vi "SphereWedgeSection.vi"(0 "Ducer":cluster{"radius":dbl, "h":dbl, "a":dbl} {"radius" format="%.2f"; "a" format="%.2f"; "h" format="%.2f"}, 2 "Rotate":dbl format="%.2f") -> (1 "thetas":dbl[](array[numeric]) format="%.2f", 4 "phis":dbl[](array[numeric]) format="%.2f", 6 "x matrix":dbl[][](array[numeric]) format="%.2f", 7 "y matrix":dbl[][](array[numeric]) format="%.2f", 8 "z matrix":dbl[][](array[numeric]) format="%.2f")   [LabVIEW 2022 SP3]
uses:
  <vilib>/Analysis/NI_AALPro.lvlib
panel:
  out "XY Graph":cluster{dbl[], dbl[]}(graph)
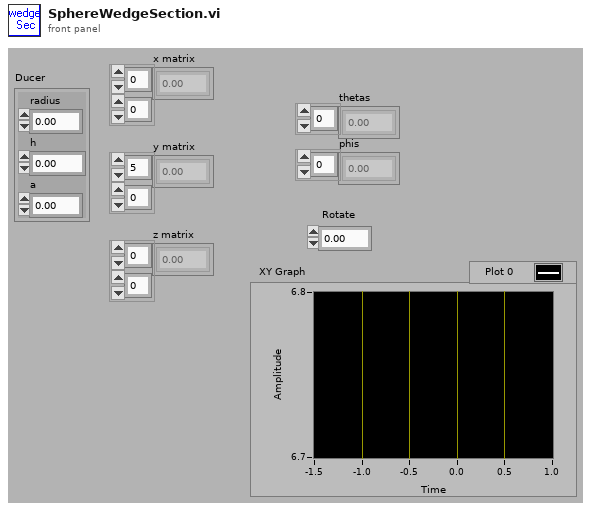
[diagram p1: front panel]
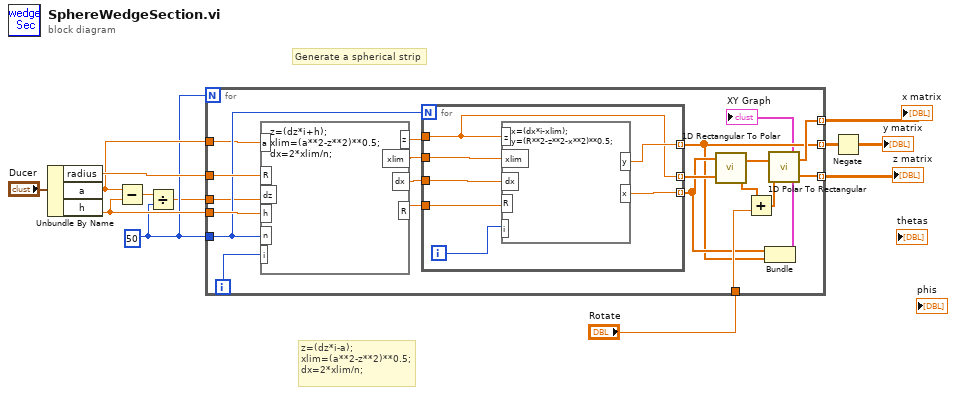
[diagram p0: block diagram]
diagram:
  w2 = 50
  # "z=(dz*i-a);\nxlim=(a**2-z**2)**0.5;\ndx=2*xlim/n;"
  # "Generate a spherical strip"
  n1 = Unbundle By Name("Ducer") -> ("radius"=w11:dbl, "a"=w5:dbl, "h"=w4:dbl)
  n2 = Subtract(x=w5, y=w4) -> (x-y=w3:dbl)
  n3 = Divide(x=w3, y=w2) -> (x/y=w1:dbl)
  n4 = for {
    N: w2 -> [_]
    tunnel: [w19] -> w10 mode=indexing
    tunnel: [w14] -> w9 mode=indexing
    tunnel: [w20] -> w8 mode=indexing
    tunnel: w11 -> [w32]
    tunnel: w4 -> [w31]
    tunnel: w2 -> [w30]
    tunnel: w5 -> [w26]
    tunnel: "Rotate" -> [w21]
    tunnel: w1 -> [w18]
    i -> [w27]
    n5 = formula code="z=(dz*i+h);\nxlim=(a**2-z**2)**0.5;\ndx=2*xlim/n;"("R"=w32, "dz"=w18, "h"=w31, "n"=w30, "i"=w27, "a"=w26) -> ("dx"=w28:dbl, "R"=w29:dbl, "xlim"=w17:dbl, "z"=w16:dbl)
    n6 = for {
      N: w30 -> [_]
      tunnel: [w39] -> w14 mode=indexing
      tunnel: [w33] -> w25 mode=indexing
      tunnel: w29 -> [w36]
      tunnel: w16 -> [w33]
      tunnel: w28 -> [w38]
      tunnel: w17 -> [w35]
      tunnel: [w34] -> w15 mode=indexing
      i -> [w37]
      n7 = formula code="x=(dx*i-xlim);\ny=(R**2-z**2-x**2)**0.5;"("dx"=w38, "xlim"=w35, "i"=w37, "R"=w36, "z"=w33) -> ("y"=w39:dbl, "x"=w34:dbl)
    }
    n8 = call <vilib>:"1D Rectangular To Polar.vi"("X"=w15, "Y"=w25) -> ("Magnitude"=w24:dbl[], "Phase"=w23:dbl[])  [unwired: 1 out]
    n9 = Add(x=w23, y=w21) -> (x+y=w22:dbl[])
    n10 = Bundle(w15, w14) -> (→"XY Graph":cluster{dbl[], dbl[]})  [unwired: 1 out]
    n11 = call <vilib>:"1D Polar To Rectangular.vi"("Magnitude"=w24, "Phase"=w22) -> ("X"=w19:dbl[], "Y"=w20:dbl[])  [unwired: 1 out]
  }
  "z matrix" <- w8
  "x matrix" <- w10
  n12 = Negate(x=w9) -> (-x=→"y matrix":dbl[][])
